vi "Read MicronConfig.vi"(8 "error in (no error)":errorcluster, 11 "MicronGRPC in":refnum<class "MicronGRPC.lvclass">) -> (0 "error out":errorcluster, 2 "MicronConfig":T1, 3 "MicronGRPC out":refnum<class "MicronGRPC.lvclass">)   [LabVIEW 2019, in "MicronGRPCGeneratedServer.lvlib" / "MicronGRPC.lvclass"]
uses:
  MicronGRPC.lvclass
  Base/Server/Service/Typedefs/MicronConfig.ctl
  MicronGRPC.lvclass/MicronGRPC.ctl
  Base/Server/Service/ServiceBase.lvclass
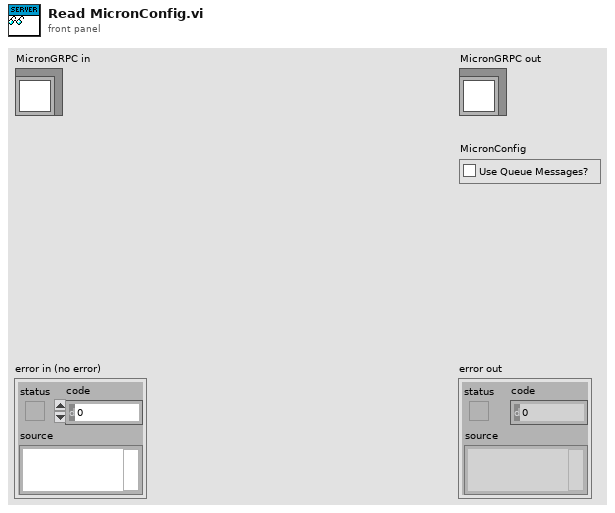
[diagram p1: front panel]
types:
  T1 = typedef "MicronServer.lvlib/ServiceBase.lvclass/MicronConfig.ctl" = cluster{"Use Queue Messages?":bool}
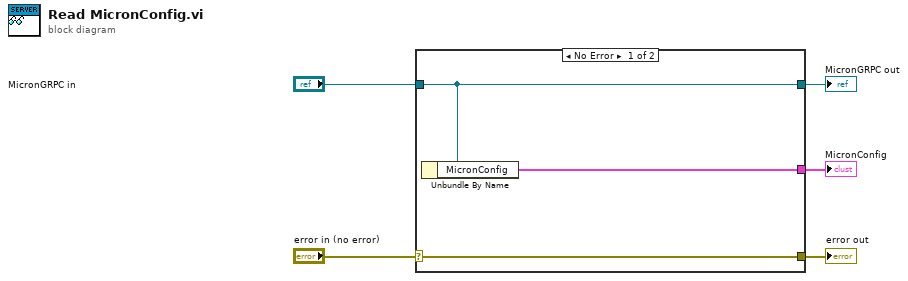
[diagram p0: block diagram]
diagram:
  n1 = case shown="No Error" "error in (no error)" {
    selector: "error in (no error)" -> [w8 w9]
    tunnel: [w8 w9] -> w4
    tunnel: [w7 w10] -> w2
    tunnel: "MicronGRPC in" -> [w7 w10]
    tunnel: [w6 _] -> w1
    frame No Error {
      n2 = Unbundle By Name(w7) -> ("MicronConfig"=w6:T1)
    }
    frame Error {
    }
  }
  "error out" <- w4
  "MicronGRPC out" <- w2
  "MicronConfig" <- w1
